vi "Send Line.vi"(8 "error in (no error)":errorcluster, 9 "Termination Char":T1=enum."\\r\\n", 10 "data":string, 11 "Serial Base in":refnum<class "Serial Base.lvclass">) -> (0 "error out":errorcluster, 2 "bytes count":u32, 3 "Serial Base out":refnum<class "Serial Base.lvclass">)   [LabVIEW 2022 SP3, in "Serial Base.lvclass"]
doc: "<b>Description</b>\nSend data string with termination character into the serial buffer and returns the byte count sent\n----------------------------------------------------------------\n<b>data</b>: data to be sent into the serial buffer\n<b>termination character</b>termination character to be added at the end of the string\nLinefeed = \\n\nCarriage return = \\r\nEnd of Line = \\r\\n"
uses:
  Serial Base.lvclass
  Termination Character--enum.ctl
  Serial Base.lvclass/Serial Base.ctl
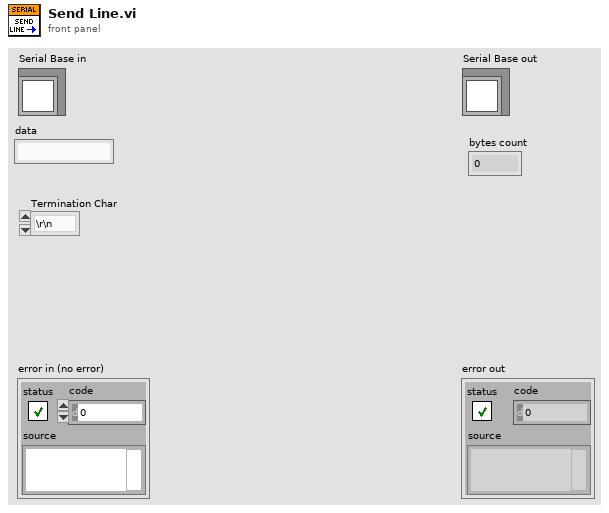
[diagram p1: front panel]
types:
  T1 = typedef "Serial Base.lvclass/Termination Character--enum.ctl" = enum16{"none", "\\r\\n", "\\r", "\\n"}
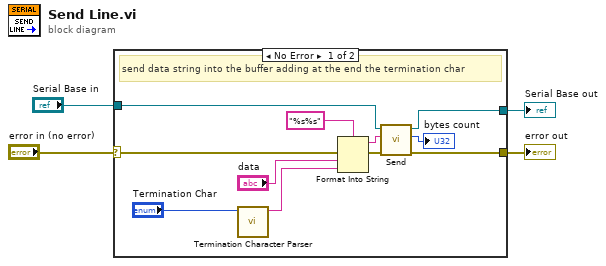
[diagram p0: block diagram]
diagram:
  n1 = case shown="No Error" "error in (no error)" {
    selector: "error in (no error)" -> [w8 w17]
    tunnel: [w13 w17] -> w3
    tunnel: [w14 w16] -> w1
    tunnel: "Serial Base in" -> [w15 w16]
    frame No Error {
      # "send data string into the buffer adding at the end the termination char"
      n2 = call "Termination Character Parser.vi"("Termination Char"="Termination Char") -> ("String"=w5:string)  [unwired: 10 in]
      n3 = Format Into String(format string="%s%s", error in=w8, "data", w5) -> (resulting string=w11:string, error out=w7:errorcluster)  [unwired: 1 in]
      n4 = call-dynamic "Send.vi"("error in (no error)"=w7, "data"=w11, "Serial Base in"=w15) -> ("error out"=w13:errorcluster, "bytes count"=→"bytes count":u32, "Serial Base out"=w14:refnum<class "Serial Base.lvclass">)  [unwired: 6 in]
    }
    frame Error {
    }
  }
  "error out" <- w3
  "Serial Base out" <- w1
